vi "Example-Find&Open&CloseDevice.vi"() -> ()   [LabVIEW 2018]
uses:
  InstrumentsPlayground.lvlib
panel:
  out "close return":i32
  in  "count 2":i32
  in  "msTimeout":i32
  out "data out":u8[](array[numeric])
  in  "读取":bool
  in  "停止":bool
  in  "count":i32
  in  "写入":bool
  in  "command":u8[](array[numeric]) format="%.0x"
  out "function return":i32
  out "error out":errorcluster caption="错误输出"
  in  "error in (no error)":errorcluster caption="错误输入（无错误）"
  out "ftHandle out":u64
  out "设备数量":u32
  in  "设备索引":i32
  out "SNs":string[](array[string])
  out "Descriptions":string[](array[string])
  # "0:success"
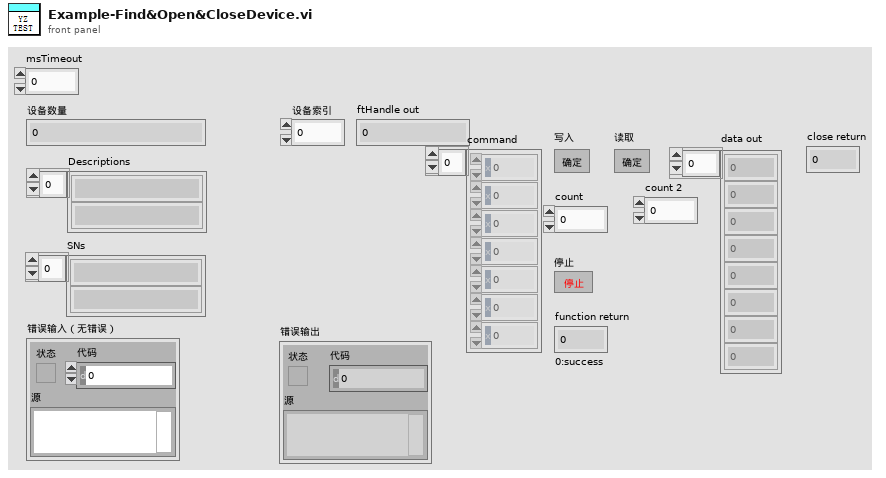
[diagram p1: front panel]
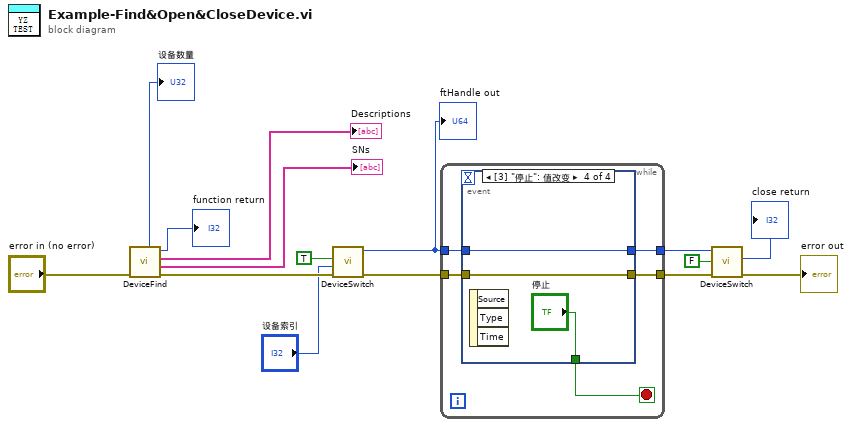
[diagram p0: block diagram]
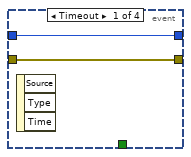
[diagram p2: hidden frame]
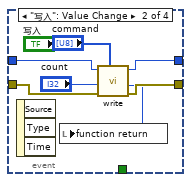
[diagram p3: hidden frame]
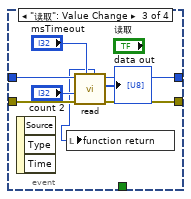
[diagram p4: hidden frame]
diagram:
  n1 = call "DeviceFind.vi"("error in (no error)"="error in (no error)") -> ("error out"=w10:errorcluster, "SNs"=→"SNs":string[], "Descriptions"=→"Descriptions":string[], "function return"=→"function return":i32, "设备数量"=→"设备数量":u32)  [unwired: 6 in]
  n2 = call "DeviceSwitch.vi"("error in (no error)"=w10, "Device Index"="设备索引", "Open"=TRUE) -> ("error out"=w9:errorcluster, "handle out"=w8:u64)  [unwired: 4 in, 3 out]
  "ftHandle out" <- w8
  n3 = while {
    tunnel: w8 -> [w20]
    tunnel: w9 -> [w19]
    tunnel: [w18] -> w6
    tunnel: [w17] -> w3
    stop <- w16 stop-if-true
    n4 = event shown="[3] \"停止\": 值改变" {
      selector: _ -> [_ _ _ _]
      dyn-events: _ -> [_ _ _ _]
      timeout: _ -> [_ _ _ _]
      tunnel: w20 -> [w21 w27 w37 w39]
      tunnel: w19 -> [w22 w26 w34 w38]
      tunnel: [w22 w25 w35 w38] -> w18
      tunnel: [w21 w24 w36 w39] -> w17
      tunnel: [_ _ _ "停止"] -> w16
      event Timeout {
        n5 = event-data() -> ()  [unwired: 1 in, 3 out]
      }
      event "写入": Value Change {
        n6 = event-data() -> ()  [unwired: 1 in, 3 out]
        n7 = call "write.vi"("command"="command", "error in (no error)"=w26, "count"="count", "handle"=w27) -> ("error out"=w25:errorcluster, "function return"=w23:i32, "handle out"=w24:u64)  [unwired: 5 in]
        n8 = local write "function return"(w23) -> ()
      }
      event "读取": Value Change {
        n9 = event-data() -> ()  [unwired: 1 in, 3 out]
        n10 = call "read.vi"("msTimeout"="msTimeout", "error in (no error)"=w34, "count"="count 2", "handle"=w37) -> ("error out"=w35:errorcluster, "data out"=→"data out":u8[], "handle out"=w36:u64, "function return"=w30:i32)  [unwired: 3 in, 1 out]
        n11 = local write "function return"(w30) -> ()
      }
      event "停止": Value Change {
        n12 = event-data() -> ()  [unwired: 1 in, 3 out]
      }
    }
  }
  n13 = call "DeviceSwitch.vi"("error in (no error)"=w6, "Open"=FALSE, "handle"=w3) -> ("error out"=→"error out":errorcluster, "function return"=→"close return":i32)  [unwired: 4 in, 3 out]
